vi "FPGA Main Default.vi"() -> ()   [LabVIEW 2014]
doc: "The myRIO v1.1 FPGA Shipping Personality. This personality contains support for:\n- 2 Analog Input Interrupt channel\n- 4 Digital Input Interrupt channel\n- 1 Timer\n- 1 Accelerometer\n- 1 Button\n- 4 LED\n- 10 Analog Input channels with 1 Sample\n- 6 Analog Output channels with 1 Sample\n- 40 Digital I/O channels with 1 Sample\n- 2 I2C channels\n- 4 Encoder channels\n- 6 PWM channels\n- 2 SPI channels"
uses:
  <vilib>/eio/EIONode/EIONode.xnode
  <vilib>/rvi/eio/common/nirviEmuTemplateMethod_errors.vi
  <vilib>/Platform/TimedLoop/XDataNode/wakeup.ctl
  <vilib>/Platform/TimedLoop/XDataNode/XDNodeRunTimeDep.lvlib
  <vilib>/Platform/TimedLoop/XDataNode/nitl_modes.ctl
  <vilib>/Platform/TimedLoop/XDataNode/timing_clust.ctl
  <vilib>/Platform/TimedLoop/XDataNode/XDataNode.xnode
  <vilib>/rvi/DataTransferAndStorage/Container/XNode/niFpgaContainer.xnode
  <vilib>/rvi/FIFO/Fifo_Resource/nirvififoEmulationWrite.vi
  <vilib>/rvi/FIFO/Fifo_Resource/nirvififoEmulationRead.vi
  <vilib>/rvi/LocalResourceManager/LocalResourceManager.xnode
  <vilib>/rvi/eio/common/nirviEmuReportErrorAndStop.vi
  <vilib>/rvi/DataTransferAndStorage/Container/Common/niFpgaContainerGetUniqueNameForEmu.vi
  <vilib>/rvi/DataTransferAndStorage/Container/Common/niFpgaContainerSetEmuInfo.vi
  Sub VIs/Utilities/Start Boolean.ctl
panel:
  in  "AO.A_0.VAL":u16
  in  "AO.A_1.VAL":u16
  in  "AO.B_0.VAL":u16
  in  "AO.B_1.VAL":u16
  out "AI.B_3.VAL":u16
  out "AI.B_2.VAL":u16
  out "AI.B_1.VAL":u16
  out "AI.B_0.VAL":u16
  out "AI.A_3.VAL":u16
  out "AI.A_2.VAL":u16
  out "AI.A_1.VAL":u16
  out "AI.A_0.VAL":u16
  out "DIO.B_7:0.IN":u8 format="%08b"
  in  "DIO.B_7:0.DIR":u8 format="%08b"
  in  "DIO.B_7:0.OUT":u8 format="%08b"
  in  "PWM.A_2.CS":u8=1
  in  "PWM.A_2.CNFG":u8=4
  out "PWM.A_2.CNTR":u16
  in  "PWM.A_2.MAX":u16=39999
  in  "PWM.A_2.CMP":u16=20000
  in  "PWM.A_1.CS":u8=1
  in  "PWM.A_1.CNFG":u8=4
  out "PWM.A_1.CNTR":u16
  in  "PWM.A_1.MAX":u16=39999
  in  "PWM.A_1.CMP":u16=20000
  in  "PWM.A_0.CS":u8=1
  in  "PWM.A_0.CNFG":u8=4
  out "PWM.A_0.CNTR":u16
  in  "PWM.A_0.CMP":u16=20000
  in  "PWM.A_0.MAX":u16=39999
  in  "SPI.A.DATO":u16
  out "SPI.A.DATI":u16
  in  "SPI.A.CNFG":u16=112
  in  "SPI.A.CNT":u16=19
  in  "SPI.B.CNT":u16=19
  in  "SPI.B.CNFG":u16=112 format="%0.0f"
  out "SPI.B.DATI":u16
  in  "SPI.B.DATO":u16
  in  "ENC.A.CNFG":u8 format="%08b"
  in  "ENC.B.CNFG":u8 format="%08b"
  out "ENC.A.CNTR":u32
  out "ENC.B.CNTR":u32
  out "ENC.A.STAT":u8 format="%08b"
  out "ENC.B.STAT":u8 format="%08b"
  in  "SPI.A.GO":T1
  out "SPI.A.STAT":u8 format="%08b"
  in  "SPI.B.GO":T1
  out "SPI.B.STAT":u8 format="%08b"
  out "I2C.B.STAT":u8 format="%08b"
  in  "I2C.B.CNTL":u8 format="%08b"
  out "I2C.A.STAT":u8 format="%08b"
  in  "I2C.A.CNTL":u8 format="%08b"
  in  "I2C.B.CNTR":u8=213
  in  "I2C.B.ADDR":u8 format="%08.0f"
  out "I2C.B.DATI":u8
  in  "I2C.B.DATO":u8
  in  "I2C.A.CNTR":u8=213
  in  "I2C.A.ADDR":u8 format="%08b"
  out "I2C.A.DATI":u8
  in  "I2C.A.DATO":u8
  in  "I2C.B.CNFG":u8=1 format="%08b"
  in  "I2C.A.CNFG":u8=1 format="%08b"
  in  "I2C.A.GO":T1
  in  "I2C.B.GO":T1
  out "SYS.AI.RDY":bool
  out "SYS.RDY":bool
  in  "PWM.B_2.CS":u8=1
  in  "PWM.B_2.CNFG":u8=4
  out "PWM.B_2.CNTR":u16
  in  "PWM.B_2.MAX":u16=39999
  in  "PWM.B_2.CMP":u16=20000
  in  "PWM.B_1.CS":u8=1
  in  "PWM.B_1.CNFG":u8=4
  out "PWM.B_1.CNTR":u16
  in  "PWM.B_1.MAX":u16=39999
  in  "PWM.B_1.CMP":u16=20000
  in  "PWM.B_0.CS":u8=1
  in  "PWM.B_0.CNFG":u8=4
  out "PWM.B_0.CNTR":u16
  in  "PWM.B_0.MAX":u16=39999
  in  "PWM.B_0.CMP":u16=20000
  out "DIO.A_7:0.IN":u8 format="%08b"
  in  "DIO.A_7:0.OUT":u8 format="%08b"
  in  "DIO.A_7:0.DIR":u8 format="%08b"
  out "DIO.C_7:0.IN":u8 format="%08b"
  in  "DIO.C_7:0.DIR":u8 format="%08b"
  in  "DIO.C_7:0.OUT":u8 format="%08b"
  out "AI.C_1.VAL":u16
  out "AI.C_0.VAL":u16
  in  "AO.C_0.VAL":u16
  in  "AO.C_1.VAL":u16
  in  "SYS.SELECTB":u8 format="%08b"
  in  "SYS.SELECTC":u8 format="%08b"
  in  "SYS.SELECTA":u8 format="%08b"
  in  "ENC.C_0.CNFG":u8 format="%08b"
  out "ENC.C_0.CNTR":u32
  out "ENC.C_0.STAT":u8 format="%08b"
  in  "ENC.C_1.CNFG":u8 format="%08b"
  out "ENC.C_1.CNTR":u32
  out "ENC.C_1.STAT":u8 format="%08b"
  in  "PWM.C_1.CS":u8=1
  in  "PWM.C_1.CNFG":u8=4
  out "PWM.C_1.CNTR":u16
  in  "PWM.C_1.CMP":u16=20000
  in  "PWM.C_1.MAX":u16=39999
  in  "PWM.C_0.CS":u8=1
  in  "PWM.C_0.CNFG":u8=4
  out "PWM.C_0.CNTR":u16
  in  "PWM.C_0.CMP":u16=20000
  in  "PWM.C_0.MAX":u16=39999
  out "DIO.A_15:8.IN":u8 format="%08b"
  in  "DIO.A_15:8.OUT":u8 format="%08b"
  in  "DIO.A_15:8.DIR":u8 format="%08b"
  out "DIO.B_15:8.IN":u8 format="%08b"
  in  "DIO.B_15:8.DIR":u8 format="%08b"
  in  "DIO.B_15:8.OUT":u8 format="%08b"
  out "AI.AudioIn_R.VAL":u16
  out "AI.AudioIn_L.VAL":u16
  in  "AO.AudioOut_R.VAL":u16
  in  "AO.AudioOut_L.VAL":u16
  in  "AO.SYS.GO":T1
  out "ACC.X.VAL":u16
  out "ACC.Y.VAL":u16
  out "SYS.ACC.RDY":bool
  out "ACC.Z.VAL":u16
  in  "DO.LED3:0":u8 format="%04b"
  out "DI.BTN":u8 format="%08b"
  out "AO.SYS.STAT":bool
  in  "AI.A.IRQ.CNFG":fxp<+,4,4> format="%.0b"
  in  "AI.A_0.THRESHOLD":u16
  in  "AI.A_1.THRESHOLD":u16
  in  "AI.A_0.IRQ.NO":u8
  in  "AI.A_1.IRQ.NO":u8
  in  "DIO.A_7:0.IRQ.ENA":fxp<+,4,4> format="%08b"
  in  "DIO.A_7:0.IRQ.RISE":fxp<+,4,4> format="%08b"
  in  "DIO.A_7:0.IRQ.FALL":fxp<+,4,4> format="%08b"
  in  "DIO.A_0.IRQ.NO":u8
  in  "DIO.A_1.IRQ.NO":u8
  in  "DIO.A_2.IRQ.NO":u8
  in  "DIO.A_3.IRQ.NO":u8
  in  "DIO.A_3.IRQ.CNT":u32
  in  "DIO.A_2.IRQ.CNT":u32
  in  "DIO.A_1.IRQ.CNT":u32
  in  "DIO.A_0.IRQ.CNT":u32
  in  "AI.A_1.HYSTERESIS":u16=17
  in  "TIMER.Write":u32
  in  "TIMER.SetTime":T1
  out "TIMER.Read":u32
  in  "SPI.A.IRQ.NO":u8=15
  in  "SPI.B.IRQ.NO":u8=15
  in  "AI.A_0.HYSTERESIS":u16=17
  in  "DI.BTN.IRQ.ENA":bool
  in  "DI.BTN.IRQ.RISE":bool
  in  "DI.BTN.IRQ.FALL":bool
  in  "DI.BTN.IRQ.CNT":u32
  in  "DI.BTN.IRQ.NO":u8
  # "System"
  # "Onboard Devices"
  # "Connector A"
  # "Connector B"
  # "Connector C"
  # "Audio Connector"
  # "Accelerometer"
  # "Analog Input"
  # "Analog Output"
  # "Digital I/O"
  # "PWM"
  # "SPI Master"
  # "Analog Input"
  # "Analog Output"
  # "Digital I/O"
  # "PWM"
  # "SPI Master"
  # "Analog Input"
  # "Analog Output"
  # "Digital I/O"
  # "Counters / PWM"
  # "Analog Input"
  # "Analog Output"
  # "IO Configuration"
  # "IO Configuration"
  # "IO Configuration"
  # "Encoders"
  # "Buttons & LEDs"
  # "Analog Interrupt"
  # "Digital Interrupt"
  # "Encoders"
  # "Encoders"
  # "FPGA Timer"
  # "I2C Master"
  # "I2C Master"
  # "Button Interrupt"
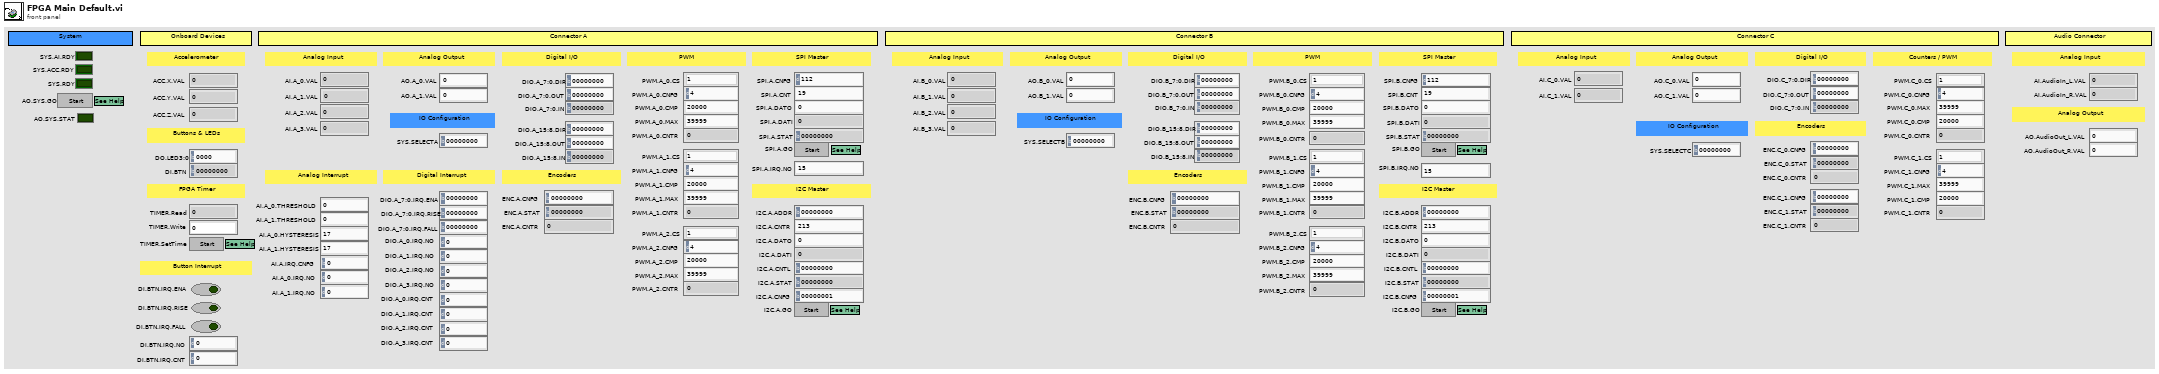
[diagram p1: front panel]
types:
  T1 = typedef "Start Boolean.ctl" = bool
  T2 = typedef "XDNodeRunTimeDep.lvlib/timing_clust.ctl" = cluster{"Expected End [f-1]":u64, "Actual End [f-1]":u64, "Finished Late? [f-1]":bool, "Expected End [i-1]":u64, "Actual End [i-1]":u64, "Finished Late? [i-1]":bool, "Expected Start [i]":u64, "Actual Start [i]":u64, "Expected Start [f]":u64, "Actual Start [f]":u64, "Source Name":string, "Structure Name":string, "Period":i64, "Deadline":i64, "Offset":i64, "Start":i64, "Priority":i32, "Timeout":i32, "Mode":T3, "Wakeup Reason":T4, "Error":errorcluster, "Source Type":string, "Secondary Source Type":string, "Global End Time":u64, "Global Start Time":u64, "Frame Duration":u64, "Iteration Duration":u64, "Assigned CPU":i32, "I/O Scan Engine Mode":u32}
  T3 = typedef "XDNodeRunTimeDep.lvlib/nitl_modes.ctl" = enum32{"No Change", "Process missed periods, maintain original phase", "Discard missed periods, maintain original phase", "Process missed periods, ignore original phase", "Discard missed periods, ignore original phase"}
  T4 = typedef "XDNodeRunTimeDep.lvlib/wakeup.ctl" = enum32{"Normal", "Aborted", "Asynchronous wakeup", "Timing source error", "Timed loop error", "Timeout"}
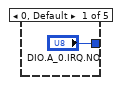
[diagram p11: hidden frame]
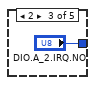
[diagram p12: hidden frame]
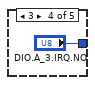
[diagram p13: hidden frame]
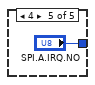
[diagram p14: hidden frame]
diagram:
  # "The Timed Loop does not allow writing the same FIFO outside the Timed Loop. Use another FIFO to push all interrupts from DIO in the Timed Loop to the IRQ Queue."
  # "The Timed Loop does not allow writing the same FIFO outside the Timed Loop. Use another FIFO to push all interrupts from Button in the Timed Loop to the IRQ Queue."
  # "The Timed Loop does not allow writing the same FIFO outside the Timed Loop. Use another FIFO to push all interrupts from DIO in the Timed Loop to the IRQ Queue."
  # "The accelerometer nodes take some time before the FPGA can first read the values. This is because it takes time to read from the accelerometer. An iteration of the While Loop will not complete until the accelerometer values have been read.\n\nAfter the completion of the first iteration of the While Loop, all indicators have valid values."
  # "The analog output nodes take some time before the FPGA write the values to the pins. The GO and STAT registers are used to handshake between the FPGA and host. When the host wants the values to be written, the host sets the GO register to TRUE. If the host reads the STAT register before setting the value of the GO register, it can wait for the value of the STAT register to invert. The value inversion tells the host that the output values have been written."
  # "The analog input nodes take some time before the FPGA can first read the values. This is because it takes time to set up the Analog-to-Digital converter (ADC) and convert the first reading. An iteration of the While Loop will not complete until all the analog input channels have been sampled.\n\nAfter the completion of the first iteration of the While Loop, all indicators have valid values."
  # "Note: On some hardware a \"ghosting effect\" may occur on any unconnected AI channels. For example, if channel AI0 is connected and channels AI1~AI7 are not connected the the value read at AI0 may be seen on indicators AI1~AI7. This is common for hardware that use a multiplexed (MUXed) Analog-to-Digital converter (ADC), because the input analog signal is used to charge a capacitor which does not discharge before the unconnected channel is read.\n\nYou can hide the \"ghosting effect\" by using an mask register. This register is used to decide when the indicator should be updated."
  # "The FPGA timer fires the interrupt request (IRQ) when TIMER.Read counts down to zero. If TIMER.Read is not zero, it counts down to one per microsecond."
  # "The only interface that sends interrupts to the RT side. Timer interrupts, analog input interrupts, digital input interrupts, and SPI interrupt share this interface.\n\nAll interrupts work in sequence. One interrupt waits until the previous interrupt request (IRQ) gets acknowledged on the RT side."
  # "NOTE: The SYS.RDY Boolean MUST exist and must become TRUE at some point. Otherwise, the myRIO VIs will not function correctly."
  # "There is some delay between the time when the FPGA code starts and the time when the analog inputs, accelerometer, and scaling values outputs are valid. If the host wants to ensure that there are valid values in theses registers it should wait for each subsystem to finish its initialization process. \n\nWhen all subsystems have finished initializinig, the SYS.RDY indicator turns true. The host can poll the SYS.RDY indicator to determine the status of the FPGA. Alternatively, the host can poll the individual SYS.xx.RDY indicators to determine the status of the individual subsystems.\n\nThis loop continues indefinitely, essentially making SYS.RDY a read-only register."
  n1 = while {
    stop <- FALSE stop-if-true
    # "Host Synchronization"
    n2 = local read "SYS.ACC.RDY"() -> (w11:bool)
    n3 = local read "SYS.AI.RDY"() -> (w13:bool)
    n4 = Compound Arithmetic op=AND(w13, w11) -> (→"SYS.RDY":bool)
  }
  n5 = while {
    stop <- FALSE stop-if-true
    # "Interrupt to RT"
    n6 = xnode ("FIFO Method Node")("Timeout"=-1) -> ("Element"=w16:u8)  [unwired: 1 in, 2 out]
    n7 = call <vilib>:"niFPGA Interrupt.vi"("Wait Until Cleared (F)"=TRUE, "IRQ Number (0)"=w16) -> ()  [unwired: 1 in]
  }
  n8 = while {
    stop <- FALSE stop-if-true
    # "Timer"
    n9 = local read "TIMER.Read"() -> (w21:u32)
    n10 = Select(t="TIMER.Write", s="TIMER.SetTime", f=w21) -> (s? t:f=w19:u32)
    n11 = case shown="Default" w19 {
      selector: w19 -> [w25 w28]
      tunnel: [w25 w26] -> w18
      frame 0 {
      }
      frame Default {
        n12 = Decrement(x=w28) -> (x-1=w27:u32)
        n13 = case shown="0" w27 {
          selector: w27 -> [w29 w32]
          tunnel: [w29 w32] -> w26
          frame Default {
          }
          frame 0 {
            w31 = u8 0  # Reserved for Timer IRQ
            n14 = xnode ("FIFO Method Node")("Element"=w31, "Timeout"=-1) -> ()  [unwired: 1 in, 2 out]
          }
        }
      }
    }
    "TIMER.Read" <- w18
    n15 = call "Loop Timer"("Count(uSec)"=u8 1 ("Count(mSec)")) -> ()  [unwired: 1 out]
  }
  n16 = xnode "VI-Defined FIFO Configuration"() -> ("FIFO Out"=w1:refnum<k21>)
  n17 = while {
    tunnel: w1 -> [w34]
    i -> [w61]
    stop <- FALSE stop-if-true
    # "Analog Input"
    n18 = xnode "FPGA I/O Node"() -> ("ConnectorA/AI0"=w39, "ConnectorA/AI1"=w38, "ConnectorA/AI2"=→"AI.A_2.VAL", "ConnectorA/AI3"=→"AI.A_3.VAL", "ConnectorB/AI0"=→"AI.B_0.VAL", "ConnectorB/AI1"=→"AI.B_1.VAL", "ConnectorB/AI2"=→"AI.B_2.VAL", "ConnectorB/AI3"=→"AI.B_3.VAL", "ConnectorC/AI0"=w55, "ConnectorC/AI1"=w54, "AudioIn/Left"=w53, "AudioIn/Right"=w52)  [unwired: 12 in, 12 out]
    "AI.A_0.VAL" <- w39
    "AI.A_1.VAL" <- w38
    n19 = Greater Than 0?(x=w61) -> (x > 0?=→"SYS.AI.RDY":bool)
    n20 = Number To Boolean Array(number="AI.A.IRQ.CNFG") -> (Boolean array=w49:bool[])
    n21 = Index Array(array=w49) -> (element #1=w47:bool, element #2=w46:bool, element #3=w44:bool, element #4=w43:bool)  [unwired: 4 in]
    n22 = To Unsigned Word Integer(number=w55) -> (unsigned 16bit integer=→"AI.C_0.VAL":u16)
    n23 = To Unsigned Word Integer(number=w54) -> (unsigned 16bit integer=→"AI.C_1.VAL":u16)
    n24 = To Unsigned Word Integer(number=w53) -> (unsigned 16bit integer=→"AI.AudioIn_L.VAL":u16)
    n25 = To Unsigned Word Integer(number=w52) -> (unsigned 16bit integer=→"AI.AudioIn_R.VAL":u16)
    n26 = call "Check AI IRQ.vi"("Hysteresis"="AI.A_1.HYSTERESIS", "FIFO In"=w34, "IRQ.Number"="AI.A_1.IRQ.NO", "Threshold"="AI.A_1.THRESHOLD", "Analog Value"=w38, "Rising Edge?"=w43, "Enable Interrupt?"=w44) -> ()  [unwired: 5 in]
    n27 = call "Check AI IRQ.vi"("Hysteresis"="AI.A_0.HYSTERESIS", "FIFO In"=w34, "IRQ.Number"="AI.A_0.IRQ.NO", "Threshold"="AI.A_0.THRESHOLD", "Analog Value"=w39, "Rising Edge?"=w46, "Enable Interrupt?"=w47) -> ()  [unwired: 5 in]
  }
  n28 = while {
    stop <- FALSE stop-if-true
    # "Analog Output"
    n29 = feedback #1(FALSE) -> (w67:bool)
    n30 = case shown="True" "AO.SYS.GO" {
      tunnel: "AO.C_0.VAL" -> [_ w89]
      tunnel: "AO.C_1.VAL" -> [_ w88]
      tunnel: "AO.A_0.VAL" -> [_ w93]
      tunnel: "AO.A_1.VAL" -> [_ w92]
      tunnel: "AO.B_0.VAL" -> [_ w91]
      tunnel: "AO.B_1.VAL" -> [_ w90]
      tunnel: "AO.AudioOut_L.VAL" -> [_ w85]
      tunnel: "AO.AudioOut_R.VAL" -> [_ w84]
      tunnel: w67 -> [w78 w81]
      tunnel: [w78 w79] -> w65
      frame False {
      }
      frame True {
        n31 = To Word Integer(number=w89) -> (16bit integer=w87:i16)
        n32 = To Word Integer(number=w88) -> (16bit integer=w86:i16)
        n33 = To Word Integer(number=w85) -> (16bit integer=w83:i16)
        n34 = To Word Integer(number=w84) -> (16bit integer=w82:i16)
        n35 = flat-sequence {
          tunnel: w93 -> [w102]
          tunnel: w92 -> [w101]
          tunnel: w91 -> [w100]
          tunnel: w90 -> [w99]
          tunnel: w87 -> [w98]
          tunnel: w86 -> [w97]
          tunnel: w83 -> [w96]
          tunnel: w82 -> [w95]
          tunnel: w81 -> [w94]
          tunnel: [w94] -> w80
          tunnel: w80 -> [w104]
          tunnel: [w103] -> w79
          frame #0 {
            n36 = xnode "FPGA I/O Node"("ConnectorA/AO0"=w102, "ConnectorA/AO1"=w101, "ConnectorB/AO0"=w100, "ConnectorB/AO1"=w99, "ConnectorC/AO0"=w98, "ConnectorC/AO1"=w97, "AudioOut/Left"=w96, "AudioOut/Right"=w95) -> ()  [unwired: 8 in, 8 out]
          }
          frame #1 {
            n37 = Not(x=w104) -> (.not. x?=w103:bool)
          }
        }
      }
    }
    "AO.SYS.STAT" <- w65
    n38 = feedback-in #1(w65) -> ()
  }
  n39 = while {
    i -> [w109]
    stop <- FALSE stop-if-true
    # "Onboard Accelerometer"
    n40 = xnode "FPGA I/O Node"() -> ("AccelerationX"=w112, "AccelerationY"=w111, "AccelerationZ"=w110)  [unwired: 3 in, 3 out]
    n41 = Greater Than 0?(x=w109) -> (x > 0?=→"SYS.ACC.RDY":bool)
    n42 = To Unsigned Word Integer(number=w112) -> (unsigned 16bit integer=→"ACC.X.VAL":u16)
    n43 = To Unsigned Word Integer(number=w111) -> (unsigned 16bit integer=→"ACC.Y.VAL":u16)
    n44 = To Unsigned Word Integer(number=w110) -> (unsigned 16bit integer=→"ACC.Z.VAL":u16)
  }
  n45 = node-c288() -> (w3:T2)  [unwired: 1 in]
  n46 = timed-loop {
    timing: w3 -> [_]
    timing-out: [_] -> w2
    stop <- _ stop-if-true
    # "Onboard DIO"
    n47 = xnode "FPGA I/O Node"() -> ("Button0"=w119)  [unwired: 1 in, 1 out]
    n48 = Number To Boolean Array(number="DO.LED3:0") -> (Boolean array=w129:bool[])
    n49 = Index Array(array=w129) -> (element #1=w128:bool, element #2=w127:bool, element #3=w126:bool, element #4=w125:bool)  [unwired: 4 in]
    n50 = call "Check DI IRQ.vi"("Debounce Ticks"=u16 40000, "Count"="DI.BTN.IRQ.CNT", "On Falling Edge?"="DI.BTN.IRQ.FALL", "On Rising Edge?"="DI.BTN.IRQ.RISE", "Enable Interrupt?"="DI.BTN.IRQ.ENA", "Digital In"=w119) -> ("Trigger?"=w120:bool)  [unwired: 5 in]
    n51 = xnode "FPGA I/O Node"("LED0"=w128, "LED1"=w127, "LED2"=w126, "LED3"=w125) -> ()  [unwired: 4 in, 4 out]
    n52 = Build Array(w119) -> (w132:void[])
    n53 = feedback #2(FALSE ("Timed Out?")) -> (w123:bool)
    n54 = Or(x=w120, y=w123) -> (x .or. y?=w121:bool)
    n55 = case shown="True" w121 {
      selector: w121 -> [w133 _]
      tunnel: [w133 w135] -> w122
      frame False {
      }
      frame True {
        n56 = xnode ("FIFO Method Node")("Element"="DI.BTN.IRQ.NO", "Timeout"=0) -> ("Timed Out?"=w135:bool)  [unwired: 1 in, 1 out]
      }
    }
    n57 = feedback-in #2(w122) -> ()
    n58 = Boolean Array To Number(Boolean array=w132) -> (number=→"DI.BTN":u8)
  }
  n59 = xnode "VI-Defined FIFO Configuration"() -> ()  [unwired: 1 out]
  n60 = while {
    stop <- FALSE stop-if-true
    # "Button SCTL Interrupt Buffer"
    n61 = feedback #3(u8 0 ("Element")) -> (w141:u8)
    n62 = feedback #4(FALSE ("Timed Out?")) -> (w145:bool)
    n63 = case shown="False" w145 {
      tunnel: [w147 w149] -> w142
      tunnel: w141 -> [_ w149]
      frame False {
        n64 = xnode ("FIFO Method Node")("Timeout"=-1) -> ("Element"=w147:u8)  [unwired: 1 in, 2 out]
      }
      frame True {
      }
    }
    n65 = feedback-in #3(w142) -> ()
    n66 = xnode ("FIFO Method Node")("Element"=w142, "Timeout"=0) -> ("Timed Out?"=w143:bool)  [unwired: 1 in, 1 out]
    n67 = feedback-in #4(w143) -> ()
  }
  n68 = node-c288(w2) -> ()
  n69 = node-c288() -> (w7:T2)  [unwired: 1 in]
  n70 = xnode "VI-Defined FIFO Configuration"() -> ()  [unwired: 1 out]
  n71 = while {
    stop <- FALSE stop-if-true
    # "Connector A SCTL Interrupt Buffer"
    n72 = feedback #5(u8 0 ("Element")) -> (w152:u8)
    n73 = feedback #6(FALSE ("Timed Out?")) -> (w156:bool)
    n74 = case shown="False" w156 {
      tunnel: [w158 w160] -> w153
      tunnel: w152 -> [_ w160]
      frame False {
        n75 = xnode ("FIFO Method Node")("Timeout"=-1) -> ("Element"=w158:u8)  [unwired: 1 in, 2 out]
      }
      frame True {
      }
    }
    n76 = feedback-in #5(w153) -> ()
    n77 = xnode ("FIFO Method Node")("Element"=w153, "Timeout"=0) -> ("Timed Out?"=w154:bool)  [unwired: 1 in, 1 out]
    n78 = feedback-in #6(w154) -> ()
  }
  n79 = timed-loop {
    timing: w7 -> [_]
    timing-out: [_] -> w6
    stop <- _ stop-if-true
    w161 = u16 5 ("Debounce Ticks")
    w162 = u8 0
    # "Trigger the interrupt at next \ntick if timeout"
    # "DIO / Encoder"
    # "DIO / I2C Master"
    # "DIO / PWM"
    # "DIO"
    # "DIO"
    # "DIO/ SPI Master"
    # "Connector A DIO"
    n80 = call "Split HDC Bank1 DIO.vi"("IN 7:0"="DIO.A_7:0.OUT") -> ("OUT 3:0"=w297:fxp<+,4,4>, "OUT 4"=w216:bool, "OUT 7:5"=w294:fxp<+,3,3>)
    n81 = call "Split HDC Bank1 DIO.vi"("IN 7:0"="DIO.A_7:0.DIR") -> ("OUT 3:0"=w296:fxp<+,4,4>, "OUT 4"=w295:bool, "OUT 7:5"=w293:fxp<+,3,3>)
    n82 = call "Split HDC Function Select.vi"("IN 7:0"="SYS.SELECTA") -> ("OUT 1:0"=w236:fxp<+,2,2>, "OUT 7"=w231:bool, "OUT 2"=w235:bool, "OUT 3"=w234:bool, "OUT 4"=w233:bool, "OUT 5"=w232:bool)
    n83 = call "DIO 4-bit.vi"("DIO0 Refnum"=refnum<k21> "ConnectorA/DIO0", "DIO1 Refnum"=refnum<k21> "ConnectorA/DIO1", "DIO2 Refnum"=refnum<k21> "ConnectorA/DIO2", "DIR 3:0"=w296, "OUT 3:0"=w297, "DIO3 Refnum"=refnum<k21> "ConnectorA/DIO3") -> ("IN 3:0"=w184:fxp<+,4,4>)  [unwired: 5 in]
    n84 = call "DIO 1-bit.vi"("DIR"=w295, "OUT"=w216, "DIO Refnum"=refnum<k21> "ConnectorA/DIO4") -> ("IN"=w183:bool)  [unwired: 8 in]
    n85 = call "DIO_SPI.vi"("DIO.2:0.OUT"=w294, "DIO.2:0.DIR"=w293, "SPI.CNT"="SPI.A.CNT", "SPI.CNFG"="SPI.A.CNFG", "SPI.DATO"="SPI.A.DATO", "SPI.GO"="SPI.A.GO", "DIO.2/SPI.MOSI Refnum"=refnum<k21> "ConnectorA/DIO7" ("DIO.2/SPI.SCLK"), "SELECT.1:0"=w236, "DIO.1/SPI.MISO Refnum"=refnum<k21> "ConnectorA/DIO6" ("DIO.1/SPI.MOSI"), "DIO.0/SPI.SCLK Refnum"=refnum<k21> "ConnectorA/DIO5" ("DIO.0/SPI.MISO")) -> ("DIO.2:0.IN"=w269:fxp<+,3,3>, "SPI.DATI"=→"SPI.A.DATI":u16, "SPI.STAT"=w169:u8)  [unwired: 7 in]
    "SPI.A.STAT" <- w169
    n86 = Number To Boolean Array(number=w169) -> (Boolean array=w171:bool[])
    n87 = Index Array(array=w171) -> (element=w170:bool)  [unwired: 1 in]
    n88 = call "Falling Edge Trigger.vi"("Signal"=w170) -> ("Trigger?"=w168:bool)
    n89 = call "Join HDC Bank1 DIO.vi"("IN 7:5"=w269, "IN 4"=w183, "IN 3:0"=w184) -> ("OUT 7:0"=→"DIO.A_7:0.IN":u8)
    n90 = Number To Boolean Array(number=w184) -> (Boolean array=w209:bool[])
    n91 = Number To Boolean Array(number="DIO.A_7:0.IRQ.ENA") -> (Boolean array=w215:bool[])
    n92 = Number To Boolean Array(number="DIO.A_7:0.IRQ.RISE") -> (Boolean array=w214:bool[])
    n93 = Number To Boolean Array(number="DIO.A_7:0.IRQ.FALL") -> (Boolean array=w213:bool[])
    n94 = call "Split HDC Bank2 DIO.vi"("IN 7:0"="DIO.A_15:8.OUT") -> ("OUT 5"=w218:bool, "OUT 7:6"=w240:fxp<+,2,2>, "OUT 4:3"=w220:fxp<+,2,2>, "OUT 2"=w222:bool, "OUT 0"=w226:bool, "OUT 1"=w225:bool)  [unwired: 2 in]
    n95 = call "Split HDC Bank2 DIO.vi"("IN 7:0"="DIO.A_15:8.DIR") -> ("OUT 5"=w217:bool, "OUT 7:6"=w239:fxp<+,2,2>, "OUT 4:3"=w219:fxp<+,2,2>, "OUT 2"=w221:bool, "OUT 0"=w224:bool, "OUT 1"=w223:bool)  [unwired: 2 in]
    n96 = Index Array(array=w209) -> (element #1=w190:bool, element #2=w205:bool, element #3=w204:bool, element #4=w203:bool)  [unwired: 4 in]
    n97 = Index Array(array=w215) -> (element #1=w208:bool, element #2=w202:bool, element #3=w201:bool, element #4=w200:bool)  [unwired: 4 in]
    n98 = Index Array(array=w214) -> (element #1=w207:bool, element #2=w199:bool, element #3=w198:bool, element #4=w197:bool)  [unwired: 4 in]
    n99 = Index Array(array=w213) -> (element #1=w206:bool, element #2=w196:bool, element #3=w195:bool, element #4=w194:bool)  [unwired: 4 in]
    n100 = call "Check DI IRQ.vi"("Debounce Ticks"=w161, "Count"="DIO.A_0.IRQ.CNT", "On Falling Edge?"=w206, "On Rising Edge?"=w207, "Enable Interrupt?"=w208, "Digital In"=w190) -> ("Trigger?"=w181:bool)  [unwired: 5 in]
    n101 = call "Check DI IRQ.vi"("Debounce Ticks"=w161, "Count"="DIO.A_1.IRQ.CNT", "On Falling Edge?"=w196, "On Rising Edge?"=w199, "Enable Interrupt?"=w202, "Digital In"=w205) -> ("Trigger?"=w180:bool)  [unwired: 5 in]
    n102 = call "Check DI IRQ.vi"("Debounce Ticks"=w161, "Count"="DIO.A_2.IRQ.CNT", "On Falling Edge?"=w195, "On Rising Edge?"=w198, "Enable Interrupt?"=w201, "Digital In"=w204) -> ("Trigger?"=w179:bool)  [unwired: 5 in]
    n103 = call "DIO_PWM.vi"("DIO.OUT"=w226, "DIO.DIR"=w224, "PWM.CS"="PWM.A_0.CS", "PWM.CNFG"="PWM.A_0.CNFG", "PWM.CMP"="PWM.A_0.CMP", "PWM.MAX"="PWM.A_0.MAX", "DIO/PWM"=refnum<k21> "ConnectorA/DIO8", "SELECT"=w235) -> ("DIO.IN"=w230:bool, "PWM.CNTR"=→"PWM.A_0.CNTR":u16)  [unwired: 10 in]
    n104 = call "DIO_PWM.vi"("DIO.OUT"=w225, "DIO.DIR"=w223, "PWM.CS"="PWM.A_1.CS", "PWM.CNFG"="PWM.A_1.CNFG", "PWM.CMP"="PWM.A_1.CMP", "PWM.MAX"="PWM.A_1.MAX", "DIO/PWM"=refnum<k21> "ConnectorA/DIO9", "SELECT"=w234) -> ("DIO.IN"=w229:bool, "PWM.CNTR"=→"PWM.A_1.CNTR":u16)  [unwired: 10 in]
    n105 = call "DIO_PWM.vi"("DIO.OUT"=w222, "DIO.DIR"=w221, "PWM.CS"="PWM.A_2.CS", "PWM.CNFG"="PWM.A_2.CNFG", "PWM.CMP"="PWM.A_2.CMP", "PWM.MAX"="PWM.A_2.MAX", "DIO/PWM"=refnum<k21> "ConnectorA/DIO10", "SELECT"=w233) -> ("DIO.IN"=w228:bool, "PWM.CNTR"=→"PWM.A_2.CNTR":u16)  [unwired: 10 in]
    n106 = call "Check DI IRQ.vi"("Debounce Ticks"=w161, "Count"="DIO.A_3.IRQ.CNT", "On Falling Edge?"=w194, "On Rising Edge?"=w197, "Enable Interrupt?"=w200, "Digital In"=w203) -> ("Trigger?"=w178:bool)  [unwired: 5 in]
    n107 = feedback #7(w162) -> (w164:u8)
    n108 = Less?(x=w164, y=4 ("x")) -> (x < y?=w166:bool)
    n109 = Increment(x=w164) -> (x+1=w165:u8)
    n110 = Select(t=w165, s=w166, f=w162) -> (s? t:f=w163:u8)
    n111 = feedback-in #7(w163) -> ()
    n112 = case shown="1" w164 {
      tunnel: ["DIO.A_0.IRQ.NO" "DIO.A_1.IRQ.NO" "DIO.A_2.IRQ.NO" "DIO.A_3.IRQ.NO" "SPI.A.IRQ.NO"] -> w193
      frame 0, Default {
      }
      frame 1 {
      }
      frame 2 {
      }
      frame 3 {
      }
      frame 4 {
      }
    }
    n113 = Build Array(w181, w180, w179, w178, w168) -> (w176:bool[])
    n114 = call "DIO_Encoder.vi"("DIO.1:0.OUT"=w220, "DIO.1:0.DIR"=w219, "QE.CNFG"="ENC.A.CNFG", "DIO.1/QE.B"=refnum<k21> "ConnectorA/DIO12", "SELECT"=w232, "DIO.0/QE.A"=refnum<k21> "ConnectorA/DIO11") -> ("DIO.1:0.IN"=w227:fxp<+,2,2>, "QE.CNTR"=→"ENC.A.CNTR":u32, "QE.STAT"=→"ENC.A.STAT":u8)  [unwired: 11 in]
    n115 = call "DIO 1-bit.vi"("DIR"=w217, "OUT"=w218, "DIO Refnum"=refnum<k21> "ConnectorA/DIO13") -> ("IN"=w182:bool)  [unwired: 8 in]
    n116 = call "DIO_I2C.vi"("DIO.1:0.OUT"=w240, "DIO.1:0.DIR"=w239, "I2C.CNFG"="I2C.A.CNFG", "I2C.CNTL"="I2C.A.CNTL", "I2C.ADDR"="I2C.A.ADDR", "I2C.DATO"="I2C.A.DATO", "DIO.1/I2C.SDA"=refnum<k21> "ConnectorA/DIO15" ("DIO.1/I2C.SCL"), "I2C.CNTR"="I2C.A.CNTR", "DIO.0/I2C.SCL"=refnum<k21> "ConnectorA/DIO14" ("DIO.0/I2C.SDA"), "Execute?"="I2C.A.GO", "SELECT"=w231) -> ("DIO.1:0.IN"=w238:fxp<+,2,2>, "I2C.DATI"=→"I2C.A.DATI":u8, "I2C.STAT"=→"I2C.A.STAT":u8)  [unwired: 6 in]
    n117 = feedback #8(bool[] [FALSE, FALSE, FALSE, FALSE, FALSE] ("initialized array")) -> (w172:bool[])
    n118 = Or(x=w176, y=w172) -> (x .or. y?=w177:bool[])
    n119 = Index Array(array=w177, index=w164) -> (element=w175:bool)
    n120 = case shown="True" w175 {
      selector: w175 -> [w298 _]
      tunnel: [w298 w299] -> w174
      tunnel: w193 -> [_ w300]
      frame False {
      }
      frame True {
        n121 = xnode ("FIFO Method Node")("Element"=w300, "Timeout"=0) -> ("Timed Out?"=w299:bool)  [unwired: 1 in, 1 out]
      }
    }
    n122 = Replace Array Subset(array=w177, new element=w174, index=w164) -> (w173:bool[])
    n123 = feedback-in #8(w173) -> ()
    n124 = call "Join HDC Bank2 DIO.vi"("IN 7:6"=w238, "IN 5"=w182, "IN 4:3"=w227, "IN 0"=w230, "IN 2"=w228, "IN 1"=w229) -> ("OUT 7:0"=→"DIO.A_15:8.IN":u8)  [unwired: 4 in]
  }
  n125 = node-c288(w6) -> ()
  n126 = node-c288() -> (w5:T2)  [unwired: 1 in]
  n127 = timed-loop {
    timing: w5 -> [_]
    timing-out: [_] -> w4
    stop <- _ stop-if-true
    # "DIO / Encoder"
    # "DIO / I2C Master"
    # "DIO / PWM"
    # "DIO"
    # "DIO"
    # "DIO/ SPI Master"
    # "Connector B DIO"
    n128 = call "Split HDC Bank1 DIO.vi"("IN 7:0"="DIO.B_7:0.OUT") -> ("OUT 3:0"=w403:fxp<+,4,4>, "OUT 4"=w401:bool, "OUT 7:5"=w399:fxp<+,3,3>)
    n129 = call "Split HDC Bank1 DIO.vi"("IN 7:0"="DIO.B_7:0.DIR") -> ("OUT 3:0"=w402:fxp<+,4,4>, "OUT 4"=w400:bool, "OUT 7:5"=w398:fxp<+,3,3>)
    n130 = call "Split HDC Function Select.vi"("IN 7:0"="SYS.SELECTB") -> ("OUT 1:0"=w375:fxp<+,2,2>, "OUT 7"=w370:bool, "OUT 2"=w374:bool, "OUT 3"=w373:bool, "OUT 4"=w372:bool, "OUT 5"=w371:bool)
    n131 = call "DIO 4-bit.vi"("DIO0 Refnum"=refnum<k21> "ConnectorB/DIO0", "DIO1 Refnum"=refnum<k21> "ConnectorB/DIO1", "DIO2 Refnum"=refnum<k21> "ConnectorB/DIO2", "DIR 3:0"=w402, "OUT 3:0"=w403, "DIO3 Refnum"=refnum<k21> "ConnectorB/DIO3") -> ("IN 3:0"=w381:fxp<+,4,4>)  [unwired: 5 in]
    n132 = call "DIO 1-bit.vi"("DIR"=w400, "OUT"=w401, "DIO Refnum"=refnum<k21> "ConnectorB/DIO4") -> ("IN"=w380:bool)  [unwired: 8 in]
    n133 = call "DIO_SPI.vi"("DIO.2:0.OUT"=w399, "DIO.2:0.DIR"=w398, "SPI.CNT"="SPI.B.CNT", "SPI.CNFG"="SPI.B.CNFG", "SPI.DATO"="SPI.B.DATO", "SPI.GO"="SPI.B.GO", "DIO.2/SPI.MOSI Refnum"=refnum<k21> "ConnectorB/DIO7" ("DIO.2/SPI.SCLK"), "SELECT.1:0"=w375, "DIO.1/SPI.MISO Refnum"=refnum<k21> "ConnectorB/DIO6" ("DIO.1/SPI.MOSI"), "DIO.0/SPI.SCLK Refnum"=refnum<k21> "ConnectorB/DIO5" ("DIO.0/SPI.MISO")) -> ("DIO.2:0.IN"=w379:fxp<+,3,3>, "SPI.DATI"=→"SPI.B.DATI":u16, "SPI.STAT"=w309:u8)  [unwired: 7 in]
    "SPI.B.STAT" <- w309
    n134 = Number To Boolean Array(number=w309) -> (Boolean array=w316:bool[])
    n135 = Index Array(array=w316) -> (element=w312:bool)  [unwired: 1 in]
    n136 = call "Falling Edge Trigger.vi"("Signal"=w312) -> ("Trigger?"=w311:bool)
    n137 = call "Join HDC Bank1 DIO.vi"("IN 7:5"=w379, "IN 4"=w380, "IN 3:0"=w381) -> ("OUT 7:0"=→"DIO.B_7:0.IN":u8)
    n138 = feedback #9(FALSE ("Trigger?")) -> (w314:bool)
    n139 = Or(x=w311, y=w314) -> (x .or. y?=w315:bool)
    n140 = case shown="True" w315 {
      selector: w315 -> [w404 _]
      tunnel: [w404 w405] -> w310
      frame False {
      }
      frame True {
        n141 = xnode ("FIFO Method Node")("Element"="SPI.B.IRQ.NO", "Timeout"=0) -> ("Timed Out?"=w405:bool)  [unwired: 1 in, 1 out]
      }
    }
    n142 = feedback-in #9(w310) -> ()
    n143 = call "Split HDC Bank2 DIO.vi"("IN 7:0"="DIO.B_15:8.OUT") -> ("OUT 5"=w327:bool, "OUT 7:6"=w378:fxp<+,2,2>, "OUT 4:3"=w328:fxp<+,2,2>, "OUT 2"=w329:bool, "OUT 0"=w331:bool, "OUT 1"=w330:bool)  [unwired: 2 in]
    n144 = call "Split HDC Bank2 DIO.vi"("IN 7:0"="DIO.B_15:8.DIR") -> ("OUT 5"=w322:bool, "OUT 7:6"=w377:fxp<+,2,2>, "OUT 4:3"=w323:fxp<+,2,2>, "OUT 2"=w324:bool, "OUT 0"=w326:bool, "OUT 1"=w325:bool)  [unwired: 2 in]
    n145 = call "DIO_PWM.vi"("DIO.OUT"=w331, "DIO.DIR"=w326, "PWM.CS"="PWM.B_0.CS", "PWM.CNFG"="PWM.B_0.CNFG", "PWM.CMP"="PWM.B_0.CMP", "PWM.MAX"="PWM.B_0.MAX", "DIO/PWM"=refnum<k21> "ConnectorB/DIO8", "SELECT"=w374) -> ("DIO.IN"=w321:bool, "PWM.CNTR"=→"PWM.B_0.CNTR":u16)  [unwired: 10 in]
    n146 = call "DIO_PWM.vi"("DIO.OUT"=w330, "DIO.DIR"=w325, "PWM.CS"="PWM.B_1.CS", "PWM.CNFG"="PWM.B_1.CNFG", "PWM.CMP"="PWM.B_1.CMP", "PWM.MAX"="PWM.B_1.MAX", "DIO/PWM"=refnum<k21> "ConnectorB/DIO9", "SELECT"=w373) -> ("DIO.IN"=w320:bool, "PWM.CNTR"=→"PWM.B_1.CNTR":u16)  [unwired: 10 in]
    n147 = call "DIO_PWM.vi"("DIO.OUT"=w329, "DIO.DIR"=w324, "PWM.CS"="PWM.B_2.CS", "PWM.CNFG"="PWM.B_2.CNFG", "PWM.CMP"="PWM.B_2.CMP", "PWM.MAX"="PWM.B_2.MAX", "DIO/PWM"=refnum<k21> "ConnectorB/DIO10", "SELECT"=w372) -> ("DIO.IN"=w319:bool, "PWM.CNTR"=→"PWM.B_2.CNTR":u16)  [unwired: 10 in]
    n148 = call "DIO_Encoder.vi"("DIO.1:0.OUT"=w328, "DIO.1:0.DIR"=w323, "QE.CNFG"="ENC.B.CNFG", "DIO.1/QE.B"=refnum<k21> "ConnectorB/DIO12", "SELECT"=w371, "DIO.0/QE.A"=refnum<k21> "ConnectorB/DIO11") -> ("DIO.1:0.IN"=w318:fxp<+,2,2>, "QE.CNTR"=→"ENC.B.CNTR":u32, "QE.STAT"=→"ENC.B.STAT":u8)  [unwired: 11 in]
    n149 = call "DIO 1-bit.vi"("DIR"=w322, "OUT"=w327, "DIO Refnum"=refnum<k21> "ConnectorB/DIO13") -> ("IN"=w317:bool)  [unwired: 8 in]
    n150 = call "DIO_I2C.vi"("DIO.1:0.OUT"=w378, "DIO.1:0.DIR"=w377, "I2C.CNFG"="I2C.B.CNFG", "I2C.CNTL"="I2C.B.CNTL", "I2C.ADDR"="I2C.B.ADDR", "I2C.DATO"="I2C.B.DATO", "DIO.1/I2C.SDA"=refnum<k21> "ConnectorB/DIO15" ("DIO.1/I2C.SCL"), "I2C.CNTR"="I2C.B.CNTR", "DIO.0/I2C.SCL"=refnum<k21> "ConnectorB/DIO14" ("DIO.0/I2C.SDA"), "Execute?"="I2C.B.GO", "SELECT"=w370) -> ("DIO.1:0.IN"=w376:fxp<+,2,2>, "I2C.DATI"=→"I2C.B.DATI":u8, "I2C.STAT"=→"I2C.B.STAT":u8)  [unwired: 6 in]
    n151 = call "Join HDC Bank2 DIO.vi"("IN 7:6"=w376, "IN 5"=w317, "IN 4:3"=w318, "IN 0"=w321, "IN 2"=w319, "IN 1"=w320) -> ("OUT 7:0"=→"DIO.B_15:8.IN":u8)  [unwired: 4 in]
  }
  n152 = xnode "VI-Defined FIFO Configuration"() -> ()  [unwired: 1 out]
  n153 = while {
    stop <- FALSE stop-if-true
    # "Connector B SCTL Interrupt Buffer"
    n154 = feedback #10(u8 0 ("Element")) -> (w412:u8)
    n155 = feedback #11(FALSE ("Timed Out?")) -> (w416:bool)
    n156 = case shown="False" w416 {
      tunnel: [w418 w420] -> w413
      tunnel: w412 -> [_ w420]
      frame False {
        n157 = xnode ("FIFO Method Node")("Timeout"=-1) -> ("Element"=w418:u8)  [unwired: 1 in, 2 out]
      }
      frame True {
      }
    }
    n158 = feedback-in #10(w413) -> ()
    n159 = xnode ("FIFO Method Node")("Element"=w413, "Timeout"=0) -> ("Timed Out?"=w414:bool)  [unwired: 1 in, 1 out]
    n160 = feedback-in #11(w414) -> ()
  }
  n161 = node-c288(w4) -> ()
  n162 = node-c288() -> (w9:T2)  [unwired: 1 in]
  n163 = timed-loop {
    timing: w9 -> [_]
    timing-out: [_] -> w8
    stop <- _ stop-if-true
    # "Connector C  DIO"
    n164 = call "Split myDAQ DIO.vi"("IN 7:0"="DIO.C_7:0.OUT") -> ("OUT 2, OUT0"=w439:fxp<+,2,2>, "OUT 1"=w438:bool, "OUT 3"=w437:bool, "OUT 7"=w434:bool, "OUT 6, OUT 4"=w436:fxp<+,2,2>, "OUT 5"=w435:bool)  [unwired: 4 in]
    n165 = call "Split myDAQ DIO.vi"("IN 7:0"="DIO.C_7:0.DIR") -> ("OUT 2, OUT0"=w433:fxp<+,2,2>, "OUT 1"=w432:bool, "OUT 3"=w431:bool, "OUT 7"=w428:bool, "OUT 6, OUT 4"=w430:fxp<+,2,2>, "OUT 5"=w429:bool)  [unwired: 4 in]
    n166 = call "Split myDAQ Function Select.vi"("IN 7:0"="SYS.SELECTC") -> ("OUT 0"=w445:bool, "OUT 1"=w444:bool, "OUT 2"=w443:bool, "OUT 3"=w442:bool)  [unwired: 2 in]
    n167 = call "DIO_Encoder.vi"("DIO.1:0.OUT"=w439, "DIO.1:0.DIR"=w433, "QE.CNFG"="ENC.C_0.CNFG", "DIO.1/QE.B"=refnum<k21> "ConnectorC/DIO2", "SELECT"=w445, "DIO.0/QE.A"=refnum<k21> "ConnectorC/DIO0") -> ("DIO.1:0.IN"=w426:fxp<+,2,2>, "QE.CNTR"=→"ENC.C_0.CNTR":u32, "QE.STAT"=→"ENC.C_0.STAT":u8)  [unwired: 11 in]
    n168 = call "DIO 1-bit.vi"("DIR"=w432, "OUT"=w438, "DIO Refnum"=refnum<k21> "ConnectorC/DIO1") -> ("IN"=w425:bool)  [unwired: 8 in]
    n169 = call "DIO_PWM.vi"("DIO.OUT"=w437, "DIO.DIR"=w431, "PWM.CS"="PWM.C_0.CS", "PWM.CNFG"="PWM.C_0.CNFG", "PWM.CMP"="PWM.C_0.CMP", "PWM.MAX"="PWM.C_0.MAX", "DIO/PWM"=refnum<k21> "ConnectorC/DIO3", "SELECT"=w444) -> ("DIO.IN"=w424:bool, "PWM.CNTR"=→"PWM.C_0.CNTR":u16)  [unwired: 10 in]
    n170 = call "DIO_Encoder.vi"("DIO.1:0.OUT"=w436, "DIO.1:0.DIR"=w430, "QE.CNFG"="ENC.C_1.CNFG", "DIO.1/QE.B"=refnum<k21> "ConnectorC/DIO6", "SELECT"=w443, "DIO.0/QE.A"=refnum<k21> "ConnectorC/DIO4") -> ("DIO.1:0.IN"=w423:fxp<+,2,2>, "QE.CNTR"=→"ENC.C_1.CNTR":u32, "QE.STAT"=→"ENC.C_1.STAT":u8)  [unwired: 11 in]
    n171 = call "DIO 1-bit.vi"("DIR"=w429, "OUT"=w435, "DIO Refnum"=refnum<k21> "ConnectorC/DIO5") -> ("IN"=w422:bool)  [unwired: 8 in]
    n172 = call "DIO_PWM.vi"("DIO.OUT"=w434, "DIO.DIR"=w428, "PWM.CS"="PWM.C_1.CS", "PWM.CNFG"="PWM.C_1.CNFG", "PWM.CMP"="PWM.C_1.CMP", "PWM.MAX"="PWM.C_1.MAX", "DIO/PWM"=refnum<k21> "ConnectorC/DIO7", "SELECT"=w442) -> ("DIO.IN"=w421:bool, "PWM.CNTR"=→"PWM.C_1.CNTR":u16)  [unwired: 10 in]
    n173 = call "Join myDAQ DIO.vi"("IN 7"=w421, "IN 5"=w422, "IN 6, IN 4"=w423, "IN 2, IN 0"=w426, "IN 3"=w424, "IN 1"=w425) -> ("IN 7:0"=→"DIO.C_7:0.IN":u8)  [unwired: 4 in]
  }
  n174 = node-c288(w8) -> ()
